vi "Autonomous Independent.vi"   [LabVIEW 2017]
doc: "This VI is called when autonomous begins, and will automatically be terminated when autonomous ends. You can carry out timed or sensor driven robot movement independently without needing to return to the caller."
uses:
  <vilib>/Rock Robotics/WPI/ThirdParty/Phoenix-LabVIEW/Motor Controller/Controls/CTRE_Phoenix_MotorControl_ControlMode.ctl
  <vilib>/Rock Robotics/Network Tables/NT Read String.vi
  <vilib>/Rock Robotics/WPI/Utilities/WPI_GetSetVariantRefNum.vi
  <vilib>/Rock Robotics/Network Tables/NT Write Numeric Array.vi
  <vilib>/Rock Robotics/WPI/Solenoid/Deprecated/WPI_SolenoidSetBool.vi
panel:
  # "Be sure to right-click and choose Data Operations>>Make Current Value default if you want to save the array values with the VI"
types:
  T1 = typedef "WPI_RobotDriveDevRef.ctl" = cluster{"DevStatus":errorcluster, "Motors[]":T2[], "Square Inputs":bool, "Max Output":dbl}
  T2 = typedef "WPI_MotorControlDeviceRef.ctl" = cluster{"DeviceStatus":errorcluster, "Type":T3, "PWM":cluster{"PWM Channel":T4, "DeadBand":T5}, "CAN":cluster{"Device Number":u8, "SetOutput VI Ref":variant, "GetOutput VI Ref":variant, "Enable VI Ref":variant, "Disable VI Ref":variant, "Data":variant}, "Invert":bool, "DIO PWM":cluster{"PWM \"Enable\" Channel":T4, "DIOChannel":T6, "PWM Rate":dbl}}
  T3 = typedef "WPI_MotorControlType.ctl" = enum16{"PWM", "CAN", "DIO PWM"}
  T4 = typedef "FPGA_DIOPWMChannel.ctl" = enum8{"PWM 0", "PWM 1", "PWM 2", "PWM 3", "PWM 4", "PWM 5", "PWM 6", "PWM 7", "PWM 8", "PWM 9", "PWM MXP 0", "PWM MXP 1", "PWM MXP 2", "PWM MXP 3", "PWM MXP 4", "PWM MXP 5", "PWM MXP 6", "PWM MXP 7", "PWM MXP 8", "PWM MXP 9", "Invalid"}
  T5 = typedef "WPI_PWMDeadband.ctl" = cluster{"Name":string, "maxPositivePwm":i32, "minPositivePwm":i32, "centerPwm":i32, "maxNegativePwm":i32, "minNegativePwm":i32, "angularRange":u16}
  T6 = typedef "FPGA_DIOChannel.ctl" = enum8{"DIO 0", "DIO 1", "DIO 2", "DIO 3", "DIO 4", "DIO 5", "DIO 6", "DIO 7", "DIO 8", "DIO 9", "DIO MXP 0", "DIO MXP 1", "DIO MXP 2", "DIO MXP 3", "DIO MXP 4", "DIO MXP 5", "DIO MXP 6", "DIO MXP 7", "DIO MXP 8", "DIO MXP 9", "DIO MXP 10", "DIO MXP 11", "DIO MXP 12", "DIO MXP 13", "DIO MXP 14", "DIO MXP 15", "SPI Port CS1", "SPI Port CS2", "SPI Port CS3", "SPI Port MISO", "SPI Port MOSI", "Invalid"}
  T7 = typedef "CTRE_Phoenix_MotorControl_ControlMode.ctl" = u16
  T8 = typedef "WPI_SolenoidDevRef.ctl" = cluster{"DevStatus":errorcluster, "Pneumatics Control Module":u8, "Forward Solenoid Channel":T9, "Reverse Solenoid Channel":T9}
  T9 = typedef "WPI_SolenoidChannel.ctl" = enum8{"Solenoid 0", "Solenoid 1", "Solenoid 2", "Solenoid 3", "Solenoid 4", "Solenoid 5", "Solenoid 6", "Solenoid 7", "Invalid"}
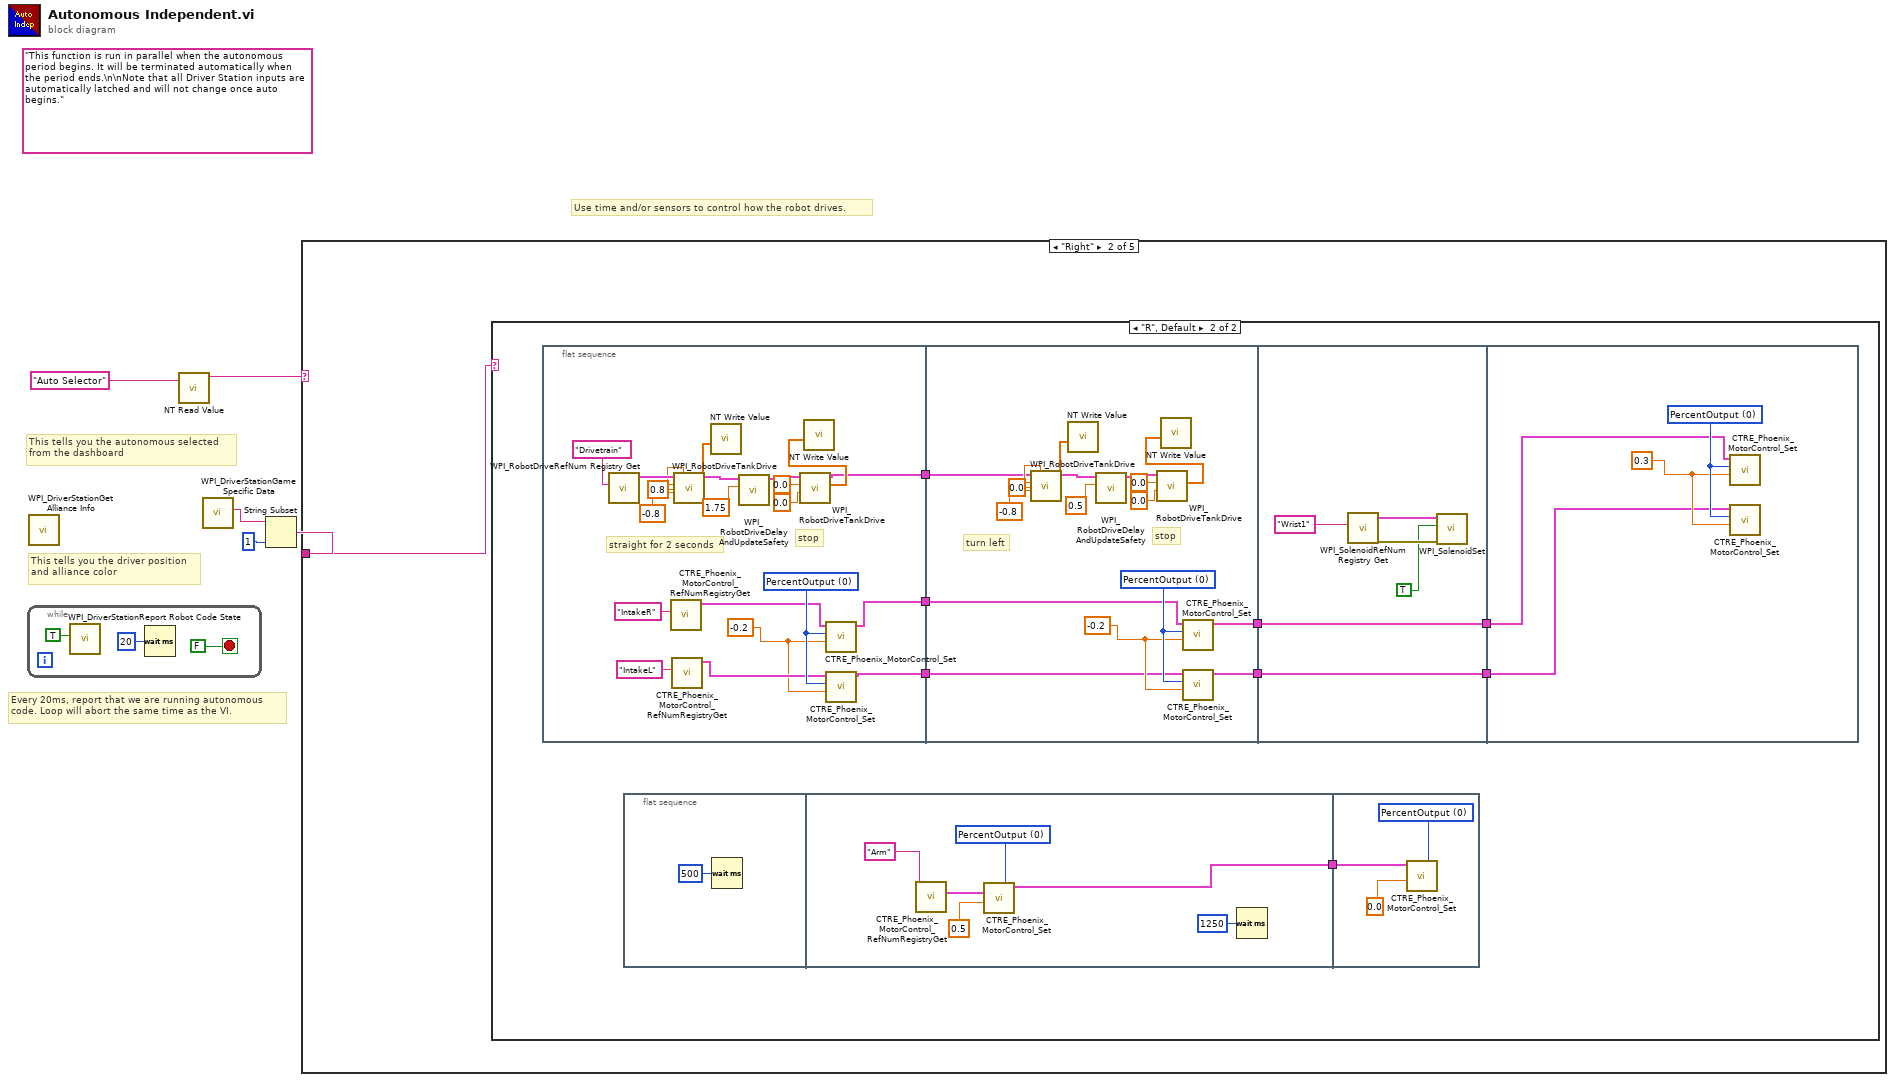
[diagram p0: block diagram]
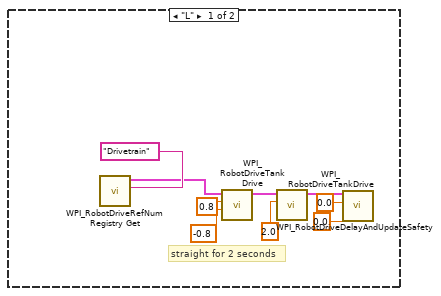
[diagram p3: hidden frame]
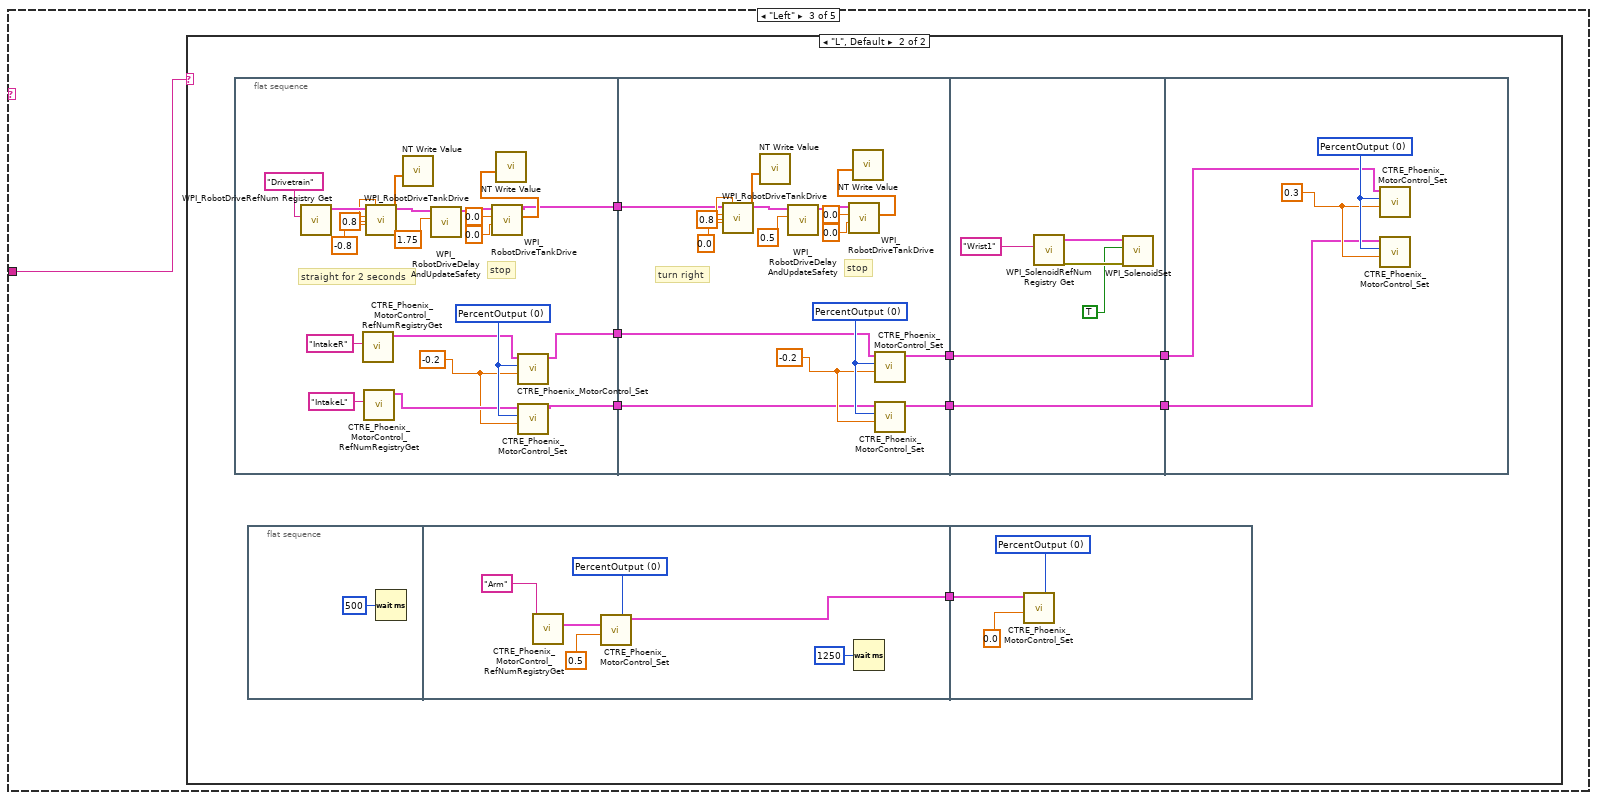
[diagram p4: hidden frame]
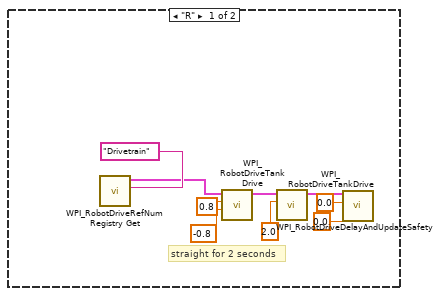
[diagram p5: hidden frame]
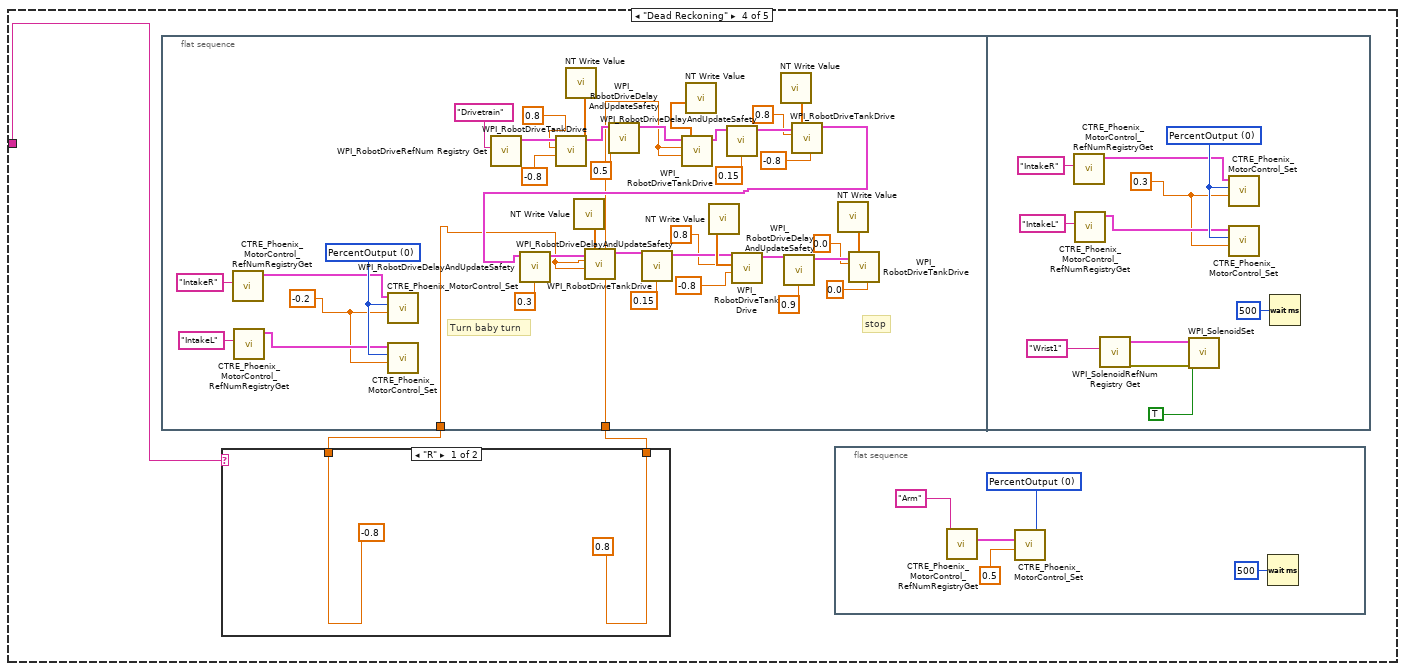
[diagram p6: hidden frame]
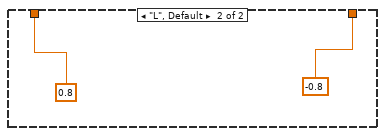
[diagram p7: hidden frame]
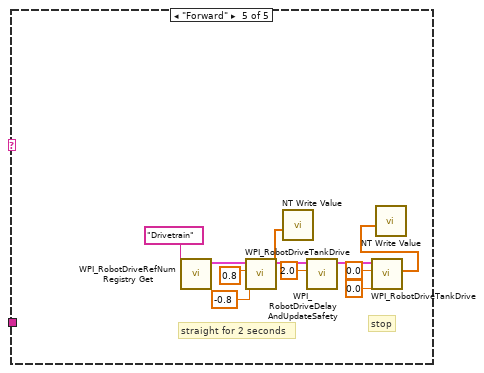
[diagram p8: hidden frame]
diagram:
  (unwired) "This function is run in parallel when the autonomous period begins. It will be terminated automatically when the period ends.\n\nNote that all Driver Station inputs are automatically latched and will not change once auto begins."
  # "This tells you the autonomous selected\nfrom the dashboard"
  # "Every 20ms, report that we are running autonomous\ncode. Loop will abort the same time as the VI."
  # "Use time and/or sensors to control how the robot drives."
  # "This tells you the driver position\nand alliance color"
  n1 = while {
    stop <- FALSE stop-if-true
    n2 = call <vilib>:"WPI_DriverStationReport Robot Code State.vi"("Autonomous"=TRUE) -> ()  [unwired: 10 in, 1 out]
    n3 = Wait (ms)(milliseconds to wait=u32 20) -> ()  [unwired: 1 out]
  }
  n4 = call <vilib>:"WPI_DriverStationGet Alliance Info.vi"() -> ()  [unwired: 12 out]
  n5 = call-poly <vilib>:"NT Read Value.vi"("Name"="Auto Selector") -> ("String"=w4:string)  [unwired: 9 in, 1 out]
  n6 = call <vilib>:"WPI_DriverStationGame Specific Data.vi"() -> ("Game Specific Data"=w1:string)  [unwired: 11 in]
  n7 = String Subset(string=w1, length (rest)=1 ("length (rest)")) -> (substring=w2:string)  [unwired: 1 in]
  n8 = case shown="\"Right\"" w4 {
    tunnel: w2 -> [_ w9 w83 w159 _]
    frame Default {
      # "You can put your main auto here, or you can right-click on the case and make any\nother frame be the default case."
      # "This is the frame that will execute if no selection is made, or if it is not recognized"
    }
    frame "Right" {
      n9 = case shown="\"R\", Default" w9 {
        frame "L" {
          # "straight for 2 seconds"
          n10 = call <vilib>:"WPI_RobotDriveRefNum Registry Get.vi"("refnum name"="Drivetrain") -> ("RobotDriveDevRef"=w16:T1)  [unwired: 9 in, 1 out]
          n11 = call <vilib>:"WPI_RobotDriveTankDrive.vi"("Right axis value"=-0.8, "Left axis value"=0.8, "RobotDriveDevRef"=w16) -> ("RobotDriveDevRef"=w17:T1)  [unwired: 6 in, 2 out]
          n12 = call <vilib>:"WPI_RobotDriveDelayAndUpdateSafety.vi"("Delay (s)"=2.0, "RobotDriveDevRef"=w17) -> ("RobotDriveDevRef 2"=w15:T1)  [unwired: 8 in, 1 out]
          n13 = call <vilib>:"WPI_RobotDriveTankDrive.vi"("Right axis value"=0.0, "Left axis value"=0.0, "RobotDriveDevRef"=w15) -> ()  [unwired: 6 in, 3 out]
        }
        frame "R", Default {
          n14 = flat-sequence {
            tunnel: [w39] -> w25
            tunnel: [w38] -> w24
            tunnel: [w37] -> w23
            tunnel: w25 -> [w61]
            tunnel: w24 -> [w60]
            tunnel: w23 -> [w59]
            tunnel: [w58] -> w21
            tunnel: [w57] -> w19
            tunnel: [w74] -> w22
            tunnel: w21 -> [w74]
            tunnel: [w73] -> w20
            tunnel: w19 -> [w73]
            tunnel: w22 -> [w80]
            tunnel: w20 -> [w79]
            frame #0 {
              w40 = -0.2
              w43 = T7 0 items=["PercentOutput"=0, "Position"=1, "Velocity"=2, "Current"=3, "Follower"=5, "MotionProfile"=6, "MotionMagic"=7, "MotionMagicArc"=8, "MotionProfileArc"=10, "Disabled"=15] ("Control Mode")
              # "stop"
              # "straight for 2 seconds"
              n15 = call <vilib>:"WPI_RobotDriveRefNum Registry Get.vi"("refnum name"="Drivetrain") -> ("RobotDriveDevRef"=w52:T1)  [unwired: 9 in, 1 out]
              n16 = call <vilib>:"CTRE_Phoenix_MotorControl_RefNumRegistryGet.vi"("refnum name"="IntakeR") -> ("PhoenixMotorControlDevRef"=w42:T2)  [unwired: 9 in, 1 out]
              n17 = call <vilib>:"CTRE_Phoenix_MotorControl_RefNumRegistryGet.vi"("refnum name"="IntakeL") -> ("PhoenixMotorControlDevRef"=w41:T2)  [unwired: 9 in, 1 out]
              n18 = call <vilib>:"WPI_RobotDriveTankDrive.vi"("Right axis value"=-0.8, "Left axis value"=0.8, "RobotDriveDevRef"=w52) -> ("Motor Values"=w55:dbl[], "RobotDriveDevRef"=w53:T1)  [unwired: 6 in, 1 out]
              n19 = call-poly <vilib>:"NT Write Value.vi"("Numeric Array"=w55) -> ()  [unwired: 10 in, 1 out]
              n20 = call <vilib>:"WPI_RobotDriveDelayAndUpdateSafety.vi"("Delay (s)"=1.75, "RobotDriveDevRef"=w53) -> ("RobotDriveDevRef 2"=w54:T1)  [unwired: 8 in, 1 out]
              n21 = call <vilib>:"WPI_RobotDriveTankDrive.vi"("Right axis value"=0.0, "Left axis value"=0.0, "RobotDriveDevRef"=w54) -> ("Motor Values"=w56:dbl[], "RobotDriveDevRef"=w39:T1)  [unwired: 6 in, 1 out]
              n22 = call-poly <vilib>:"NT Write Value.vi"("Numeric Array"=w56) -> ()  [unwired: 10 in, 1 out]
              n23 = call <vilib>:"CTRE_Phoenix_MotorControl_Set.vi"("Output"=w40, "Control Mode"=w43, "PhoenixMotorControlDevRef"=w42) -> ("PhoenixMotorControlDevRef"=w38:T2)  [unwired: 7 in, 1 out]
              n24 = call <vilib>:"CTRE_Phoenix_MotorControl_Set.vi"("Output"=w40, "Control Mode"=w43, "PhoenixMotorControlDevRef"=w41) -> ("PhoenixMotorControlDevRef"=w37:T2)  [unwired: 7 in, 1 out]
            }
            frame #1 {
              w62 = -0.2
              w63 = T7 0 items=["PercentOutput"=0, "Position"=1, "Velocity"=2, "Current"=3, "Follower"=5, "MotionProfile"=6, "MotionMagic"=7, "MotionMagicArc"=8, "MotionProfileArc"=10, "Disabled"=15] ("Control Mode")
              # "stop"
              # "turn left"
              n25 = call <vilib>:"WPI_RobotDriveTankDrive.vi"("Right axis value"=-0.8, "Left axis value"=0.0, "RobotDriveDevRef"=w61) -> ("Motor Values"=w71:dbl[], "RobotDriveDevRef"=w69:T1)  [unwired: 6 in, 1 out]
              n26 = call-poly <vilib>:"NT Write Value.vi"("Numeric Array"=w71) -> ()  [unwired: 10 in, 1 out]
              n27 = call <vilib>:"WPI_RobotDriveDelayAndUpdateSafety.vi"("Delay (s)"=0.5, "RobotDriveDevRef"=w69) -> ("RobotDriveDevRef 2"=w70:T1)  [unwired: 8 in, 1 out]
              n28 = call <vilib>:"WPI_RobotDriveTankDrive.vi"("Right axis value"=0.0, "Left axis value"=0.0, "RobotDriveDevRef"=w70) -> ("Motor Values"=w72:dbl[])  [unwired: 6 in, 2 out]
              n29 = call-poly <vilib>:"NT Write Value.vi"("Numeric Array"=w72) -> ()  [unwired: 10 in, 1 out]
              n30 = call <vilib>:"CTRE_Phoenix_MotorControl_Set.vi"("Output"=w62, "Control Mode"=w63, "PhoenixMotorControlDevRef"=w60) -> ("PhoenixMotorControlDevRef"=w58:T2)  [unwired: 7 in, 1 out]
              n31 = call <vilib>:"CTRE_Phoenix_MotorControl_Set.vi"("Output"=w62, "Control Mode"=w63, "PhoenixMotorControlDevRef"=w59) -> ("PhoenixMotorControlDevRef"=w57:T2)  [unwired: 7 in, 1 out]
            }
            frame #2 {
              n32 = call <vilib>:"WPI_SolenoidRefNum Registry Get.vi"("refnum name"="Wrist1") -> ("error out"=w78:errorcluster, "SolenoidDevRef"=w77:T8)  [unwired: 9 in]
              n33 = call-poly <vilib>:"WPI_SolenoidSet.vi"("error in (no error)"=w78, "Value"=TRUE, "SolenoidDevRef"=w77) -> ()  [unwired: 7 in, 2 out]
            }
            frame #3 {
              w81 = 0.3
              w82 = T7 0 items=["PercentOutput"=0, "Position"=1, "Velocity"=2, "Current"=3, "Follower"=5, "MotionProfile"=6, "MotionMagic"=7, "MotionMagicArc"=8, "MotionProfileArc"=10, "Disabled"=15] ("Control Mode")
              n34 = call <vilib>:"CTRE_Phoenix_MotorControl_Set.vi"("Output"=w81, "Control Mode"=w82, "PhoenixMotorControlDevRef"=w80) -> ()  [unwired: 7 in, 2 out]
              n35 = call <vilib>:"CTRE_Phoenix_MotorControl_Set.vi"("Output"=w81, "Control Mode"=w82, "PhoenixMotorControlDevRef"=w79) -> ()  [unwired: 7 in, 2 out]
            }
          }
          n36 = flat-sequence {
            tunnel: [w28] -> w26
            tunnel: w26 -> [w34]
            frame #0 {
              n37 = Wait (ms)(milliseconds to wait=u32 500) -> ()  [unwired: 1 out]
            }
            frame #1 {
              w31 = T7 0 items=["PercentOutput"=0, "Position"=1, "Velocity"=2, "Current"=3, "Follower"=5, "MotionProfile"=6, "MotionMagic"=7, "MotionMagicArc"=8, "MotionProfileArc"=10, "Disabled"=15] ("Control Mode")
              n38 = call <vilib>:"CTRE_Phoenix_MotorControl_RefNumRegistryGet.vi"("refnum name"="Arm") -> ("PhoenixMotorControlDevRef"=w32:T2)  [unwired: 9 in, 1 out]
              n39 = call <vilib>:"CTRE_Phoenix_MotorControl_Set.vi"("Output"=0.5, "Control Mode"=w31, "PhoenixMotorControlDevRef"=w32) -> ("PhoenixMotorControlDevRef"=w28:T2)  [unwired: 7 in, 1 out]
              n40 = Wait (ms)(milliseconds to wait=u32 1250) -> ()  [unwired: 1 out]
            }
            frame #2 {
              w36 = T7 0 items=["PercentOutput"=0, "Position"=1, "Velocity"=2, "Current"=3, "Follower"=5, "MotionProfile"=6, "MotionMagic"=7, "MotionMagicArc"=8, "MotionProfileArc"=10, "Disabled"=15] ("Control Mode")
              n41 = call <vilib>:"CTRE_Phoenix_MotorControl_Set.vi"("Output"=0.0, "Control Mode"=w36, "PhoenixMotorControlDevRef"=w34) -> ()  [unwired: 7 in, 2 out]
            }
          }
        }
      }
    }
    frame "Left" {
      n42 = case shown="\"L\", Default" w83 {
        frame "R" {
          # "straight for 2 seconds"
          n43 = call <vilib>:"WPI_RobotDriveRefNum Registry Get.vi"("refnum name"="Drivetrain") -> ("RobotDriveDevRef"=w90:T1)  [unwired: 9 in, 1 out]
          n44 = call <vilib>:"WPI_RobotDriveTankDrive.vi"("Right axis value"=-0.8, "Left axis value"=0.8, "RobotDriveDevRef"=w90) -> ("RobotDriveDevRef"=w91:T1)  [unwired: 6 in, 2 out]
          n45 = call <vilib>:"WPI_RobotDriveDelayAndUpdateSafety.vi"("Delay (s)"=2.0, "RobotDriveDevRef"=w91) -> ("RobotDriveDevRef 2"=w89:T1)  [unwired: 8 in, 1 out]
          n46 = call <vilib>:"WPI_RobotDriveTankDrive.vi"("Right axis value"=0.0, "Left axis value"=0.0, "RobotDriveDevRef"=w89) -> ()  [unwired: 6 in, 3 out]
        }
        frame "L", Default {
          n47 = flat-sequence {
            tunnel: [w113] -> w99
            tunnel: [w112] -> w98
            tunnel: [w111] -> w93
            tunnel: w99 -> [w135]
            tunnel: w98 -> [w134]
            tunnel: [w133] -> w96
            tunnel: [w132] -> w94
            tunnel: w93 -> [w131]
            tunnel: [w148] -> w97
            tunnel: w96 -> [w148]
            tunnel: [w147] -> w95
            tunnel: w94 -> [w147]
            tunnel: w97 -> [w154]
            tunnel: w95 -> [w153]
            frame #0 {
              w114 = -0.2
              w117 = T7 0 items=["PercentOutput"=0, "Position"=1, "Velocity"=2, "Current"=3, "Follower"=5, "MotionProfile"=6, "MotionMagic"=7, "MotionMagicArc"=8, "MotionProfileArc"=10, "Disabled"=15] ("Control Mode")
              # "stop"
              # "straight for 2 seconds"
              n48 = call <vilib>:"WPI_RobotDriveRefNum Registry Get.vi"("refnum name"="Drivetrain") -> ("RobotDriveDevRef"=w126:T1)  [unwired: 9 in, 1 out]
              n49 = call <vilib>:"CTRE_Phoenix_MotorControl_RefNumRegistryGet.vi"("refnum name"="IntakeR") -> ("PhoenixMotorControlDevRef"=w116:T2)  [unwired: 9 in, 1 out]
              n50 = call <vilib>:"CTRE_Phoenix_MotorControl_RefNumRegistryGet.vi"("refnum name"="IntakeL") -> ("PhoenixMotorControlDevRef"=w115:T2)  [unwired: 9 in, 1 out]
              n51 = call <vilib>:"WPI_RobotDriveTankDrive.vi"("Right axis value"=-0.8, "Left axis value"=0.8, "RobotDriveDevRef"=w126) -> ("Motor Values"=w129:dbl[], "RobotDriveDevRef"=w127:T1)  [unwired: 6 in, 1 out]
              n52 = call-poly <vilib>:"NT Write Value.vi"("Numeric Array"=w129) -> ()  [unwired: 10 in, 1 out]
              n53 = call <vilib>:"WPI_RobotDriveDelayAndUpdateSafety.vi"("Delay (s)"=1.75, "RobotDriveDevRef"=w127) -> ("RobotDriveDevRef 2"=w128:T1)  [unwired: 8 in, 1 out]
              n54 = call <vilib>:"WPI_RobotDriveTankDrive.vi"("Right axis value"=0.0, "Left axis value"=0.0, "RobotDriveDevRef"=w128) -> ("Motor Values"=w130:dbl[], "RobotDriveDevRef"=w111:T1)  [unwired: 6 in, 1 out]
              n55 = call-poly <vilib>:"NT Write Value.vi"("Numeric Array"=w130) -> ()  [unwired: 10 in, 1 out]
              n56 = call <vilib>:"CTRE_Phoenix_MotorControl_Set.vi"("Output"=w114, "Control Mode"=w117, "PhoenixMotorControlDevRef"=w116) -> ("PhoenixMotorControlDevRef"=w113:T2)  [unwired: 7 in, 1 out]
              n57 = call <vilib>:"CTRE_Phoenix_MotorControl_Set.vi"("Output"=w114, "Control Mode"=w117, "PhoenixMotorControlDevRef"=w115) -> ("PhoenixMotorControlDevRef"=w112:T2)  [unwired: 7 in, 1 out]
            }
            frame #1 {
              w136 = -0.2
              w137 = T7 0 items=["PercentOutput"=0, "Position"=1, "Velocity"=2, "Current"=3, "Follower"=5, "MotionProfile"=6, "MotionMagic"=7, "MotionMagicArc"=8, "MotionProfileArc"=10, "Disabled"=15] ("Control Mode")
              # "stop"
              # "turn right"
              n58 = call <vilib>:"WPI_RobotDriveTankDrive.vi"("Right axis value"=0.0, "Left axis value"=0.8, "RobotDriveDevRef"=w131) -> ("Motor Values"=w145:dbl[], "RobotDriveDevRef"=w143:T1)  [unwired: 6 in, 1 out]
              n59 = call-poly <vilib>:"NT Write Value.vi"("Numeric Array"=w145) -> ()  [unwired: 10 in, 1 out]
              n60 = call <vilib>:"WPI_RobotDriveDelayAndUpdateSafety.vi"("Delay (s)"=0.5, "RobotDriveDevRef"=w143) -> ("RobotDriveDevRef 2"=w144:T1)  [unwired: 8 in, 1 out]
              n61 = call <vilib>:"WPI_RobotDriveTankDrive.vi"("Right axis value"=0.0, "Left axis value"=0.0, "RobotDriveDevRef"=w144) -> ("Motor Values"=w146:dbl[])  [unwired: 6 in, 2 out]
              n62 = call-poly <vilib>:"NT Write Value.vi"("Numeric Array"=w146) -> ()  [unwired: 10 in, 1 out]
              n63 = call <vilib>:"CTRE_Phoenix_MotorControl_Set.vi"("Output"=w136, "Control Mode"=w137, "PhoenixMotorControlDevRef"=w135) -> ("PhoenixMotorControlDevRef"=w132:T2)  [unwired: 7 in, 1 out]
              n64 = call <vilib>:"CTRE_Phoenix_MotorControl_Set.vi"("Output"=w136, "Control Mode"=w137, "PhoenixMotorControlDevRef"=w134) -> ("PhoenixMotorControlDevRef"=w133:T2)  [unwired: 7 in, 1 out]
            }
            frame #2 {
              n65 = call <vilib>:"WPI_SolenoidRefNum Registry Get.vi"("refnum name"="Wrist1") -> ("error out"=w152:errorcluster, "SolenoidDevRef"=w151:T8)  [unwired: 9 in]
              n66 = call-poly <vilib>:"WPI_SolenoidSet.vi"("error in (no error)"=w152, "Value"=TRUE, "SolenoidDevRef"=w151) -> ()  [unwired: 7 in, 2 out]
            }
            frame #3 {
              w155 = 0.3
              w156 = T7 0 items=["PercentOutput"=0, "Position"=1, "Velocity"=2, "Current"=3, "Follower"=5, "MotionProfile"=6, "MotionMagic"=7, "MotionMagicArc"=8, "MotionProfileArc"=10, "Disabled"=15] ("Control Mode")
              n67 = call <vilib>:"CTRE_Phoenix_MotorControl_Set.vi"("Output"=w155, "Control Mode"=w156, "PhoenixMotorControlDevRef"=w153) -> ()  [unwired: 7 in, 2 out]
              n68 = call <vilib>:"CTRE_Phoenix_MotorControl_Set.vi"("Output"=w155, "Control Mode"=w156, "PhoenixMotorControlDevRef"=w154) -> ()  [unwired: 7 in, 2 out]
            }
          }
          n69 = flat-sequence {
            tunnel: [w102] -> w100
            tunnel: w100 -> [w108]
            frame #0 {
              n70 = Wait (ms)(milliseconds to wait=u32 500) -> ()  [unwired: 1 out]
            }
            frame #1 {
              w105 = T7 0 items=["PercentOutput"=0, "Position"=1, "Velocity"=2, "Current"=3, "Follower"=5, "MotionProfile"=6, "MotionMagic"=7, "MotionMagicArc"=8, "MotionProfileArc"=10, "Disabled"=15] ("Control Mode")
              n71 = call <vilib>:"CTRE_Phoenix_MotorControl_RefNumRegistryGet.vi"("refnum name"="Arm") -> ("PhoenixMotorControlDevRef"=w106:T2)  [unwired: 9 in, 1 out]
              n72 = call <vilib>:"CTRE_Phoenix_MotorControl_Set.vi"("Output"=0.5, "Control Mode"=w105, "PhoenixMotorControlDevRef"=w106) -> ("PhoenixMotorControlDevRef"=w102:T2)  [unwired: 7 in, 1 out]
              n73 = Wait (ms)(milliseconds to wait=u32 1250) -> ()  [unwired: 1 out]
            }
            frame #2 {
              w110 = T7 0 items=["PercentOutput"=0, "Position"=1, "Velocity"=2, "Current"=3, "Follower"=5, "MotionProfile"=6, "MotionMagic"=7, "MotionMagicArc"=8, "MotionProfileArc"=10, "Disabled"=15] ("Control Mode")
              n74 = call <vilib>:"CTRE_Phoenix_MotorControl_Set.vi"("Output"=0.0, "Control Mode"=w110, "PhoenixMotorControlDevRef"=w108) -> ()  [unwired: 7 in, 2 out]
            }
          }
        }
      }
    }
    frame "Dead Reckoning" {
      n75 = flat-sequence {
        tunnel: w158 -> [w166]
        tunnel: w157 -> [w165]
        frame #0 {
          w167 = -0.2
          w170 = T7 0 items=["PercentOutput"=0, "Position"=1, "Velocity"=2, "Current"=3, "Follower"=5, "MotionProfile"=6, "MotionMagic"=7, "MotionMagicArc"=8, "MotionProfileArc"=10, "Disabled"=15] ("Control Mode")
          # "stop"
          # "Turn baby turn"
          n76 = call <vilib>:"CTRE_Phoenix_MotorControl_RefNumRegistryGet.vi"("refnum name"="IntakeR") -> ("PhoenixMotorControlDevRef"=w169:T2)  [unwired: 9 in, 1 out]
          n77 = call <vilib>:"CTRE_Phoenix_MotorControl_RefNumRegistryGet.vi"("refnum name"="IntakeL") -> ("PhoenixMotorControlDevRef"=w168:T2)  [unwired: 9 in, 1 out]
          n78 = call <vilib>:"CTRE_Phoenix_MotorControl_Set.vi"("Output"=w167, "Control Mode"=w170, "PhoenixMotorControlDevRef"=w169) -> ()  [unwired: 7 in, 2 out]
          n79 = call <vilib>:"CTRE_Phoenix_MotorControl_Set.vi"("Output"=w167, "Control Mode"=w170, "PhoenixMotorControlDevRef"=w168) -> ()  [unwired: 7 in, 2 out]
          n80 = call <vilib>:"WPI_RobotDriveRefNum Registry Get.vi"("refnum name"="Drivetrain") -> ("RobotDriveDevRef"=w199:T1)  [unwired: 9 in, 1 out]
          n81 = call <vilib>:"WPI_RobotDriveTankDrive.vi"("Right axis value"=-0.8, "Left axis value"=0.8, "RobotDriveDevRef"=w199) -> ("Motor Values"=w202:dbl[], "RobotDriveDevRef"=w200:T1)  [unwired: 6 in, 1 out]
          n82 = call-poly <vilib>:"NT Write Value.vi"("Numeric Array"=w202) -> ()  [unwired: 10 in, 1 out]
          n83 = call <vilib>:"WPI_RobotDriveDelayAndUpdateSafety.vi"("Delay (s)"=0.5, "RobotDriveDevRef"=w200) -> ("RobotDriveDevRef 2"=w201:T1)  [unwired: 8 in, 1 out]
          n84 = call <vilib>:"WPI_RobotDriveTankDrive.vi"("Right axis value"=w166, "Left axis value"=w166, "RobotDriveDevRef"=w201) -> ("Motor Values"=w203:dbl[], "RobotDriveDevRef"=w189:T1)  [unwired: 6 in, 1 out]
          n85 = call-poly <vilib>:"NT Write Value.vi"("Numeric Array"=w203) -> ()  [unwired: 10 in, 1 out]
          n86 = call <vilib>:"WPI_RobotDriveDelayAndUpdateSafety.vi"("Delay (s)"=0.15, "RobotDriveDevRef"=w189) -> ("RobotDriveDevRef 2"=w193:T1)  [unwired: 8 in, 1 out]
          n87 = call <vilib>:"WPI_RobotDriveTankDrive.vi"("Right axis value"=-0.8, "Left axis value"=0.8, "RobotDriveDevRef"=w193) -> ("Motor Values"=w194:dbl[], "RobotDriveDevRef"=w185:T1)  [unwired: 6 in, 1 out]
          n88 = call <vilib>:"WPI_RobotDriveDelayAndUpdateSafety.vi"("Delay (s)"=0.3, "RobotDriveDevRef"=w185) -> ("RobotDriveDevRef 2"=w187:T1)  [unwired: 8 in, 1 out]
          n89 = call <vilib>:"WPI_RobotDriveTankDrive.vi"("Right axis value"=w165, "Left axis value"=w165, "RobotDriveDevRef"=w187) -> ("Motor Values"=w188:dbl[], "RobotDriveDevRef"=w179:T1)  [unwired: 6 in, 1 out]
          n90 = call-poly <vilib>:"NT Write Value.vi"("Numeric Array"=w188) -> ()  [unwired: 10 in, 1 out]
          n91 = call <vilib>:"WPI_RobotDriveDelayAndUpdateSafety.vi"("Delay (s)"=0.15, "RobotDriveDevRef"=w179) -> ("RobotDriveDevRef 2"=w183:T1)  [unwired: 8 in, 1 out]
          n92 = call <vilib>:"WPI_RobotDriveTankDrive.vi"("Right axis value"=-0.8, "Left axis value"=0.8, "RobotDriveDevRef"=w183) -> ("Motor Values"=w184:dbl[], "RobotDriveDevRef"=w173:T1)  [unwired: 6 in, 1 out]
          n93 = call-poly <vilib>:"NT Write Value.vi"("Numeric Array"=w184) -> ()  [unwired: 10 in, 1 out]
          n94 = call-poly <vilib>:"NT Write Value.vi"("Numeric Array"=w194) -> ()  [unwired: 10 in, 1 out]
          n95 = call <vilib>:"WPI_RobotDriveDelayAndUpdateSafety.vi"("Delay (s)"=0.9, "RobotDriveDevRef"=w173) -> ("RobotDriveDevRef 2"=w177:T1)  [unwired: 8 in, 1 out]
          n96 = call <vilib>:"WPI_RobotDriveTankDrive.vi"("Right axis value"=0.0, "Left axis value"=0.0, "RobotDriveDevRef"=w177) -> ("Motor Values"=w178:dbl[])  [unwired: 6 in, 2 out]
          n97 = call-poly <vilib>:"NT Write Value.vi"("Numeric Array"=w178) -> ()  [unwired: 10 in, 1 out]
        }
        frame #1 {
          w209 = 0.3
          w212 = T7 0 items=["PercentOutput"=0, "Position"=1, "Velocity"=2, "Current"=3, "Follower"=5, "MotionProfile"=6, "MotionMagic"=7, "MotionMagicArc"=8, "MotionProfileArc"=10, "Disabled"=15] ("Control Mode")
          n98 = call <vilib>:"CTRE_Phoenix_MotorControl_RefNumRegistryGet.vi"("refnum name"="IntakeR") -> ("PhoenixMotorControlDevRef"=w211:T2)  [unwired: 9 in, 1 out]
          n99 = call <vilib>:"CTRE_Phoenix_MotorControl_RefNumRegistryGet.vi"("refnum name"="IntakeL") -> ("PhoenixMotorControlDevRef"=w210:T2)  [unwired: 9 in, 1 out]
          n100 = call <vilib>:"WPI_SolenoidRefNum Registry Get.vi"("refnum name"="Wrist1") -> ("error out"=w207:errorcluster, "SolenoidDevRef"=w208:T8)  [unwired: 9 in]
          n101 = call-poly <vilib>:"WPI_SolenoidSet.vi"("error in (no error)"=w207, "Value"=TRUE, "SolenoidDevRef"=w208) -> ()  [unwired: 7 in, 2 out]
          n102 = call <vilib>:"CTRE_Phoenix_MotorControl_Set.vi"("Output"=w209, "Control Mode"=w212, "PhoenixMotorControlDevRef"=w211) -> ()  [unwired: 7 in, 2 out]
          n103 = call <vilib>:"CTRE_Phoenix_MotorControl_Set.vi"("Output"=w209, "Control Mode"=w212, "PhoenixMotorControlDevRef"=w210) -> ()  [unwired: 7 in, 2 out]
          n104 = Wait (ms)(milliseconds to wait=u32 500) -> ()  [unwired: 1 out]
        }
      }
      n105 = case shown="\"R\"" w159 {
        tunnel: [0.8 -0.8 ("Left axis value")] -> w158
        tunnel: [-0.8 0.8 ("Left axis value")] -> w157
        frame "R" {
        }
        frame "L", Default {
        }
      }
      n106 = flat-sequence {
        frame #0 {
          w162 = T7 0 items=["PercentOutput"=0, "Position"=1, "Velocity"=2, "Current"=3, "Follower"=5, "MotionProfile"=6, "MotionMagic"=7, "MotionMagicArc"=8, "MotionProfileArc"=10, "Disabled"=15] ("Control Mode")
          n107 = call <vilib>:"CTRE_Phoenix_MotorControl_RefNumRegistryGet.vi"("refnum name"="Arm") -> ("PhoenixMotorControlDevRef"=w163:T2)  [unwired: 9 in, 1 out]
          n108 = call <vilib>:"CTRE_Phoenix_MotorControl_Set.vi"("Output"=0.5, "Control Mode"=w162, "PhoenixMotorControlDevRef"=w163) -> ()  [unwired: 7 in, 2 out]
          n109 = Wait (ms)(milliseconds to wait=u32 500) -> ()  [unwired: 1 out]
        }
      }
    }
    frame "Forward" {
      # "stop"
      # "straight for 2 seconds"
      n110 = call <vilib>:"WPI_RobotDriveRefNum Registry Get.vi"("refnum name"="Drivetrain") -> ("RobotDriveDevRef"=w228:T1)  [unwired: 9 in, 1 out]
      n111 = call <vilib>:"WPI_RobotDriveTankDrive.vi"("Right axis value"=-0.8, "Left axis value"=0.8, "RobotDriveDevRef"=w228) -> ("Motor Values"=w220:dbl[], "RobotDriveDevRef"=w225:T1)  [unwired: 6 in, 1 out]
      n112 = call-poly <vilib>:"NT Write Value.vi"("Numeric Array"=w220) -> ()  [unwired: 10 in, 1 out]
      n113 = call <vilib>:"WPI_RobotDriveDelayAndUpdateSafety.vi"("Delay (s)"=2.0, "RobotDriveDevRef"=w225) -> ("RobotDriveDevRef 2"=w223:T1)  [unwired: 8 in, 1 out]
      n114 = call <vilib>:"WPI_RobotDriveTankDrive.vi"("Right axis value"=0.0, "Left axis value"=0.0, "RobotDriveDevRef"=w223) -> ("Motor Values"=w219:dbl[])  [unwired: 6 in, 2 out]
      n115 = call-poly <vilib>:"NT Write Value.vi"("Numeric Array"=w219) -> ()  [unwired: 10 in, 1 out]
    }
  }
